vi "Get Base Command.vi"(8 "error in (no error)":errorcluster, 11 "Measure in":refnum<class "Measure.lvclass">) -> (0 "error out":errorcluster, 2 "Base Command":string, 3 "Measure out":refnum<class "Measure.lvclass">)   [LabVIEW 2023, in "HAF.lvlib" / "Measure.lvclass"]
doc: "Returns the base command whch is used to build up the overall command string – parameters will be added to this as necessary.  The framework will add the line terminator \\n.\n\nSubclasses MUST override this member and must not add a line terminator on the end of the command; on this class an error is returned."
uses:
  Measure.lvclass
  Measure.lvclass/Measure.ctl
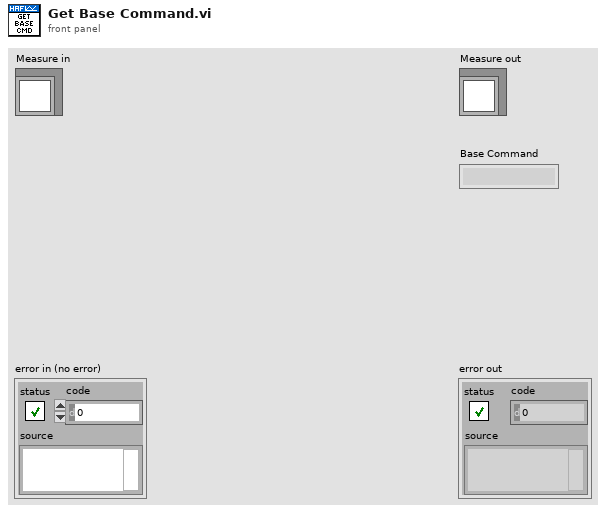
[diagram p1: front panel]
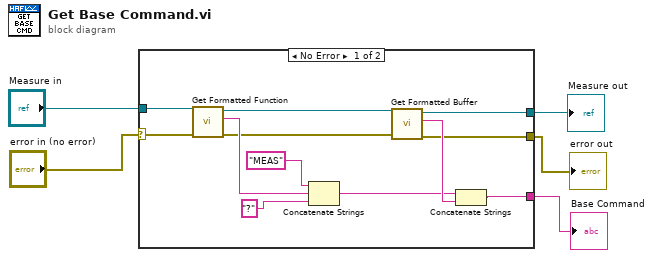
[diagram p0: block diagram]
diagram:
  n1 = case shown="No Error" "error in (no error)" {
    selector: "error in (no error)" -> [w16 w18]
    tunnel: [w8 w19] -> w2
    tunnel: "Measure in" -> [w17 w19]
    tunnel: [w7 w18] -> w1
    tunnel: [w6 _] -> w3
    frame No Error {
      n2 = call-dynamic "Get Formatted Function.vi"("error in (no error)"=w16, "Measure in"=w17) -> ("error out"=w11:errorcluster, "Function"=w15:string, "Measure out"=w12:refnum<class "Measure.lvclass">)  [unwired: 7 in]
      n3 = Concatenate Strings("MEAS" ("string"), w15, "?" ("string")) -> (w9:string)
      n4 = call-dynamic "Get Formatted Buffer.vi"("error in (no error)"=w11, "Measure in"=w12) -> ("error out"=w7:errorcluster, "Buffer Name"=w10:string, "Measure out"=w8:refnum<class "Measure.lvclass">)  [unwired: 7 in]
      n5 = Concatenate Strings(w9, w10) -> (w6:string)
    }
    frame Error {
    }
  }
  "error out" <- w1
  "Measure out" <- w2
  "Base Command" <- w3
